vi "AdvancedCounterSub.vi"(4 "Reset Counter":bool, 5 "Init Counter Value":i16, 6 "Enable HW Gate":bool, 7 "Ticks to Filter":i16, 8 "Count Direction":enum16{"Rising", "Falling"}(ring), 9 "Edge":T1(ring), 10 "Gate Signal":bool, 11 "Input Signal":bool) -> (1 "Counter Reset?":bool, 3 "Counter Out":i16)   [LabVIEW 2020]
uses:
  <vilib>/rvi/Emulation/niFpgaSctlEmulationGetInTimedLoop.vi
  <vilib>/rvi/Emulation/niFpgaProcessEmulError.vi
panel:
  out "Output Filtered Signal":bool
  out "Input Signal (Out)":bool
  out "Bucket Out":i16
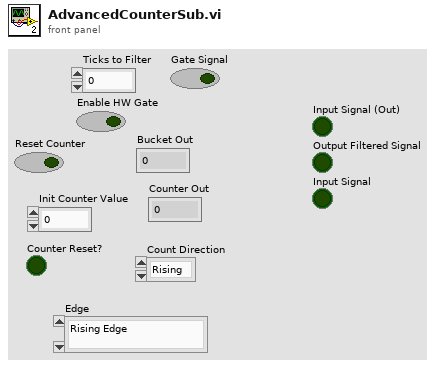
[diagram p1: front panel]
types:
  T1 = enum16{"Rising Edge", "Falling Edge", "Rising AND Falling"}
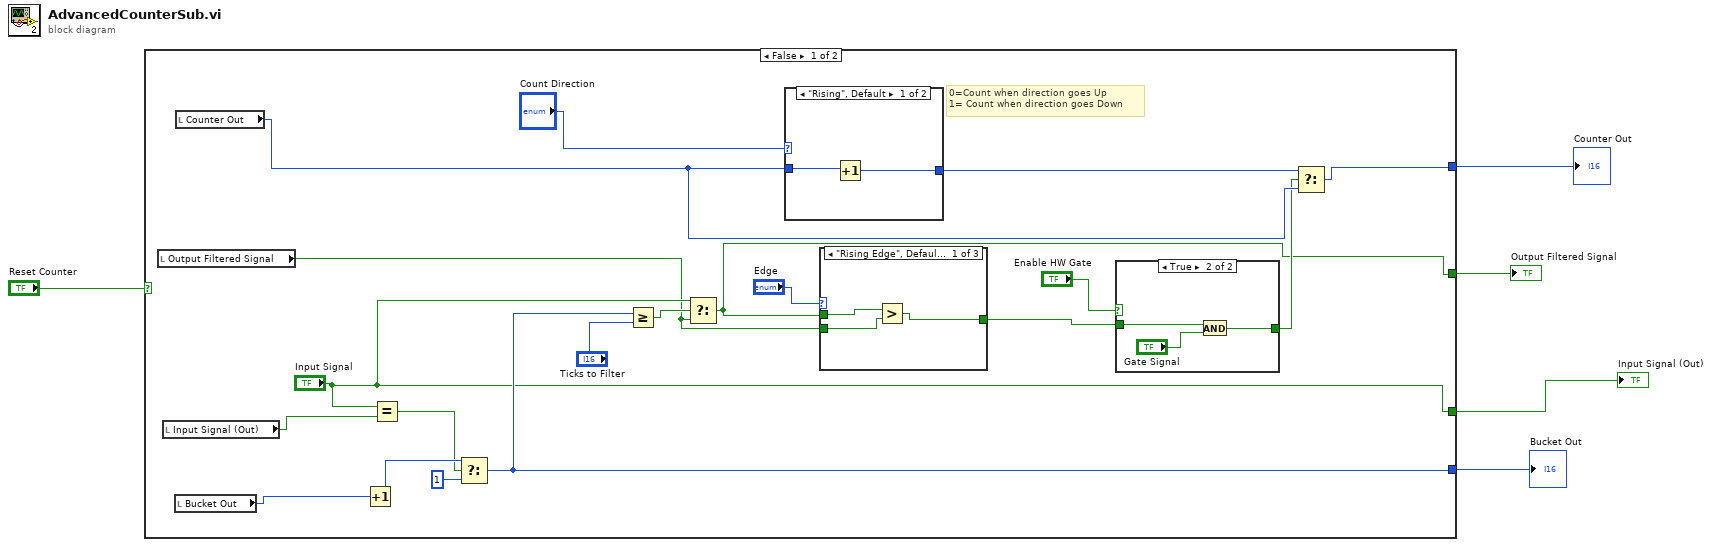
[diagram p0: block diagram]
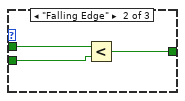
[diagram p3: hidden frame]
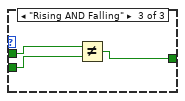
[diagram p4: hidden frame]
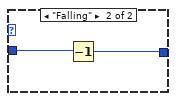
[diagram p5: hidden frame]
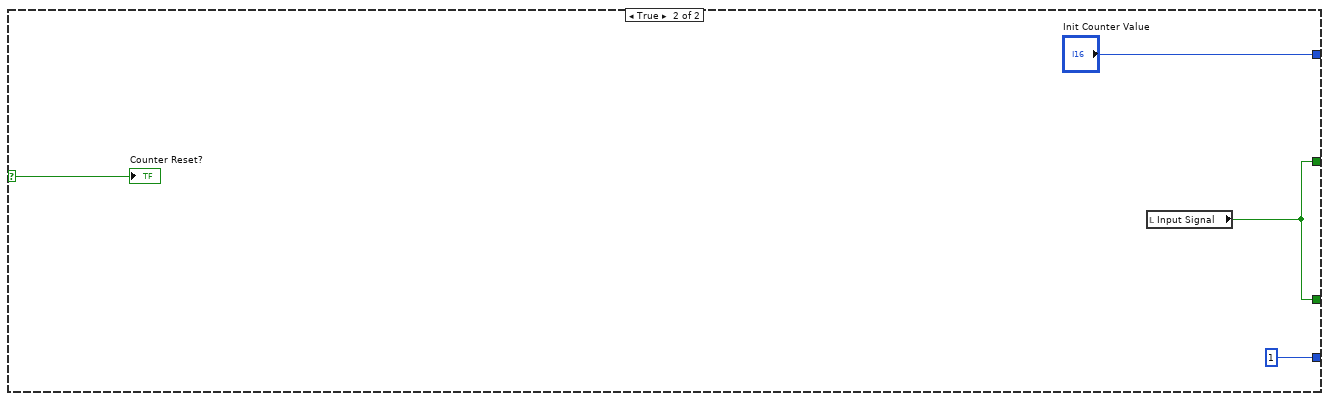
[diagram p6: hidden frame]
diagram:
  n1 = case shown="False" "Reset Counter" {
    selector: "Reset Counter" -> [_ w45]
    tunnel: [w23 "Init Counter Value"] -> w4
    tunnel: [w16 i16 1] -> w3
    tunnel: ["Input Signal" w42] -> w2
    tunnel: [w6 w42] -> w1
    frame False {
      # "0=Count when direction goes Up\n1= Count when direction goes Down"
      n2 = local read "Output Filtered Signal"() -> (w11:bool)
      n3 = local read "Input Signal (Out)"() -> (w21:bool)
      n4 = local read "Bucket Out"() -> (w20:i16)
      n5 = local read "Counter Out"() -> (w22:i16)
      n6 = Increment(x=w20) -> (x+1=w19:i16)
      n7 = Equal?(x="Input Signal", y=w21) -> (x = y?=w17:bool)
      n8 = Select(t=w19, s=w17, f=i16 1) -> (s? t:f=w16:i16)
      n9 = Greater Or Equal?(x=w16, y="Ticks to Filter") -> (x >= y?=w13:bool)
      n10 = Select(t="Input Signal", s=w13, f=w11) -> (s? t:f=w6:bool)
      n11 = case shown="\"Rising\", Default" "Count Direction" {
        tunnel: w22 -> [w39 w41]
        tunnel: [w38 w40] -> w24
        frame "Rising", Default {
          n12 = Increment(x=w39) -> (x+1=w38:i16)
        }
        frame "Falling" {
          n13 = Decrement(x=w41) -> (x-1=w40:i16)
        }
      }
      n14 = case shown="\"Rising Edge\", Default" "Edge" {
        tunnel: w11 -> [w31 w33 w37]
        tunnel: w6 -> [w30 w34 w36]
        tunnel: [w29 w32 w35] -> w9
        frame "Rising Edge", Default {
          n15 = Greater?(x=w30, y=w31) -> (0:w29:bool)
        }
        frame "Falling Edge" {
          n16 = Less?(x=w34, y=w33) -> (x < y?=w32:bool)
        }
        frame "Rising AND Falling" {
          n17 = Not Equal?(x=w36, y=w37) -> (x != y?=w35:bool)
        }
      }
      n18 = case shown="True" "Enable HW Gate" {
        tunnel: w9 -> [w25 w28]
        tunnel: [w25 w26] -> w8
        frame False {
        }
        frame True {
          n19 = And(x=w28, y="Gate Signal") -> (x .and. y?=w26:bool)
        }
      }
      n20 = Select(t=w24, s=w8, f=w22) -> (s? t:f=w23:i16)
    }
    frame True {
      n21 = local read "Input Signal"() -> (w42:bool)
      "Counter Reset?" <- w45
    }
  }
  "Counter Out" <- w4
  "Bucket Out" <- w3
  "Input Signal (Out)" <- w2
  "Output Filtered Signal" <- w1
